vi "State_Machine.vi"(8 "error in (no error)":errorcluster caption="entrée d'erreur (pas d'erreur)", 11 "Flash_AVRDUDE en entrée":refnum<class "Flash_STM32.lvclass">) -> (0 "error out":errorcluster caption="sortie d'erreur", 2 "Json_String":string, 3 "Flash_AVRDUDE en sortie":refnum<class "Flash_STM32.lvclass">)   [LabVIEW 2020, in "Library Test.lvlib" / "Flash_STM32.lvclass"]
uses:
  Flash_STM32.lvclass
  C:/Users/ngarcin/OneDrive - Altyor/Standard TB/Class/Test/Test (Default)/Test (Default).lvclass
  Flash_STM32.lvclass/Flash_STM32.ctl
panel:
  out "String In progress":string
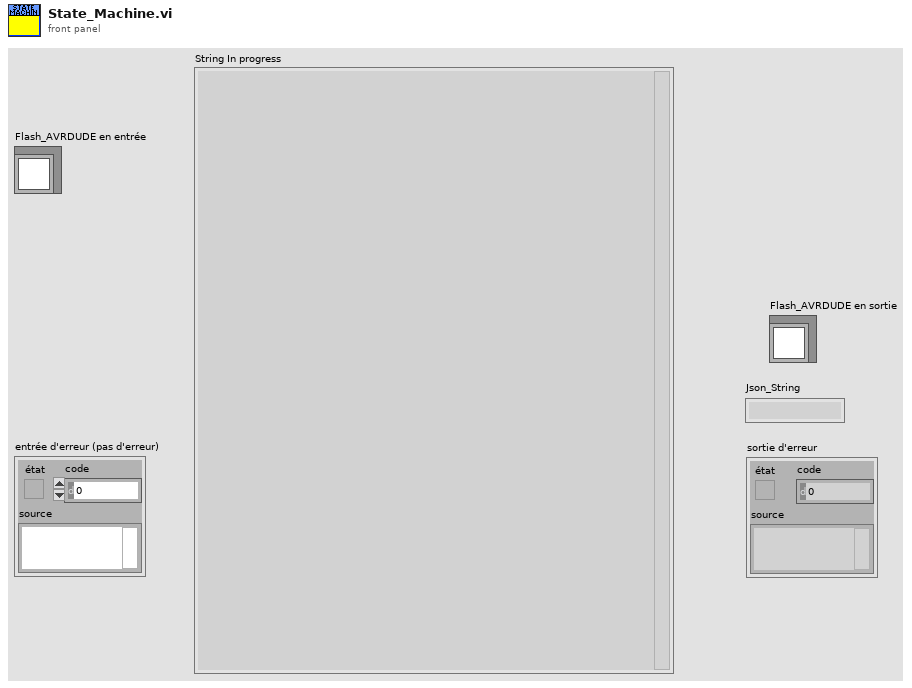
[diagram p1: front panel]
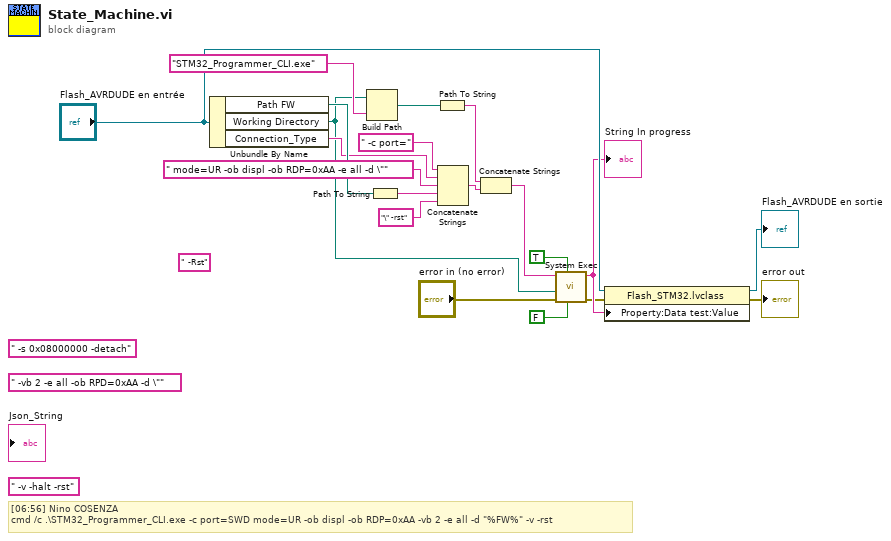
[diagram p0: block diagram]
diagram:
  (unwired) " -Rst" ("FileName")
  (unwired) " -s 0x08000000 -detach" ("chaîne")
  (unwired) " -v -halt -rst" ("FileName")
  (unwired) " -vb 2 -e all -ob RPD=0xAA -d \"" ("FileName")
  # "[06:56] Nino COSENZA\ncmd /c .\\STM32_Programmer_CLI.exe -c port=SWD mode=UR -ob displ -ob RDP=0xAA -vb 2 -e all -d \"%FW%\" -v -rst"
  n1 = Unbundle By Name("Flash_AVRDUDE en entrée") -> ("Path FW"=w15:path, "Working Directory"=w3:path, "Connection_Type"=w5:string)
  n2 = Build Path(base path=w3, name or relative path="STM32_Programmer_CLI.exe" ("nom ou chemin relatif")) -> (appended path=w20:path)
  n3 = Path To String(path=w15) -> (string=w8:string)
  n4 = Path To String(path=w20) -> (string=w7:string)
  n5 = Concatenate Strings(" -c port=" ("FileName"), w5, " mode=UR -ob displ -ob RDP=0xAA -e all -d \"" ("FileName"), w8, "\" -rst" ("chaîne")) -> (w17:string)
  n6 = Concatenate Strings(w7, w17) -> (w16:string)
  n7 = call <vilib>:"System Exec.vi"("run minimized? (F)"=FALSE, "wait until completion? (T)"=TRUE, "error in (no error)"="error in (no error)", "working directory"=w3, "command line"=w16) -> ("error out"=w1:errorcluster, "standard output"=w2:string)  [unwired: 3 in, 2 out]
  "String In progress" <- w2
  n8 = property class="Flash_STM32.lvclass"(reference="Flash_AVRDUDE en entrée", error in=w1, "Property:Data test:Value"=w2) -> (reference out=→"Flash_AVRDUDE en sortie":refnum<class "Flash_STM32.lvclass">, error out=→"error out":errorcluster)
